vi "Set Output.vi"(8 "error in (no error)":errorcluster, 10 "Output value":refnum<class "Mag Lab Result.lvclass">, 11 "Mag Lab Hardware in":refnum<class "Mag Lab Hardware.lvclass">) -> (0 "error out":errorcluster, 2 "Actual output value":refnum<class "Mag Lab Result.lvclass">, 3 "Mag Lab Hardware out":refnum<class "Mag Lab Hardware.lvclass">)   [LabVIEW 2015, in "Mag Lab Hardware.lvclass"]
uses:
  Mag Lab Hardware.lvclass
  Mag Lab Result/Mag Lab Result.lvclass
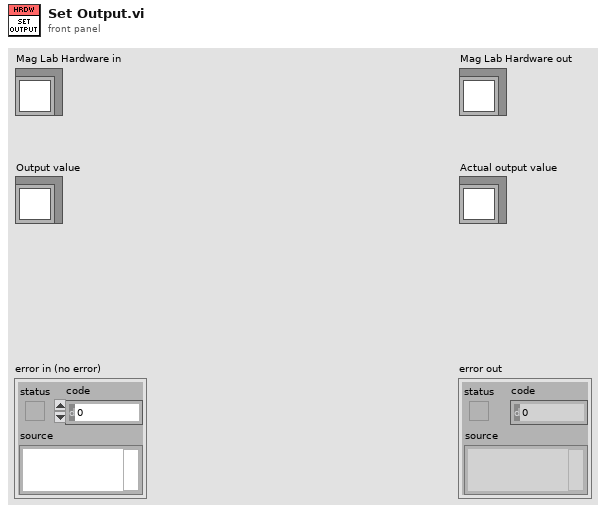
[diagram p1: front panel]
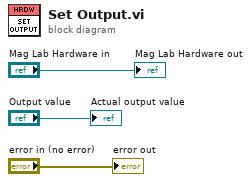
[diagram p0: block diagram]
diagram:
  "error out" <- "error in (no error)"
  "Mag Lab Hardware out" <- "Mag Lab Hardware in"
  "Actual output value" <- "Output value"
